vi "u32_to_u8[].vi"(11 "data_in":u32) -> (3 "arr_out":u8[](array[numeric]))   [LabVIEW 2021]
panel:
  out "*(type *) &x":u8[](array[numeric])
  out "reversed array":u8[](array[numeric])
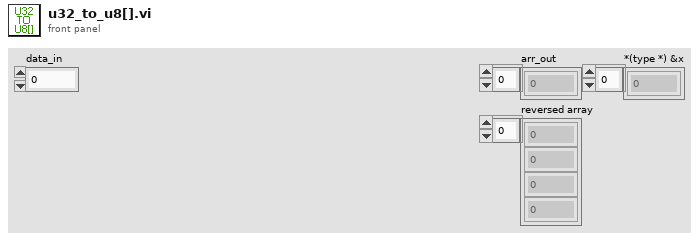
[diagram p1: front panel]
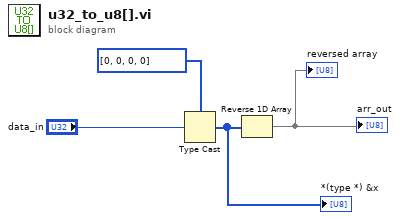
[diagram p0: block diagram]
diagram:
  n1 = Type Cast(type=u8[] [0, 0, 0, 0], x="data_in") -> (*(type *) &x=w2:u8[])
  "*(type *) &x" <- w2
  n2 = Reverse 1D Array(array=w2) -> (reversed array=→"arr_out" →"reversed array":u8[])
